vi "Schema Update.vi"(8 "error in (no error)":errorcluster, 10 "Schema":string, 11 "Signal Analysis in":refnum<class "Signal Analysis.lvclass">) -> (0 "error out":errorcluster, 3 "Signal Analysis out":refnum<class "Signal Analysis.lvclass">)   [LabVIEW 2023, in "Data Analysis.lvlib" / "Signal Analysis.lvlib" / "Signal Analysis.lvclass"]
uses:
  Signal Analysis.lvclass
  Signal Analysis.lvclass/Signal Analysis.ctl
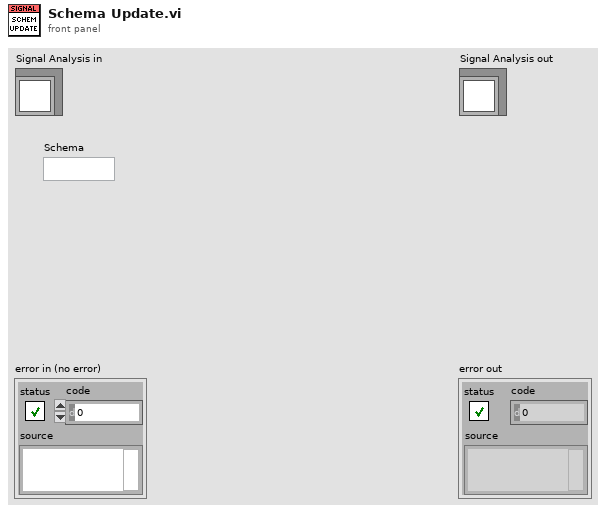
[diagram p1: front panel]
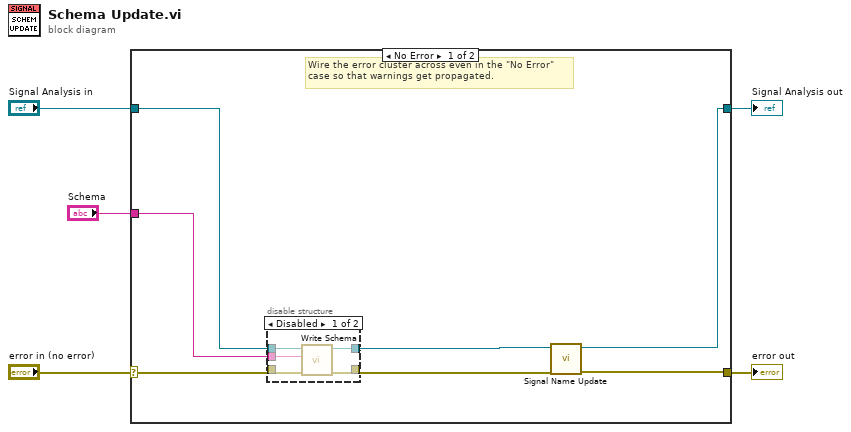
[diagram p0: block diagram]
diagram:
  n1 = case shown="No Error" "error in (no error)" {
    selector: "error in (no error)" -> [w11 w21]
    tunnel: [w6 w21] -> w4
    tunnel: [w8 w20] -> w2
    tunnel: "Signal Analysis in" -> [w12 w20]
    tunnel: "Schema" -> [w10 _]
    frame No Error {
      # "Wire the error cluster across even in the \"No Error\"\ncase so that warnings get propagated."
      n2 = disable-structure shown="Disabled" {
        disable-tunnel: w12 -> [w17 w19]
        disable-tunnel: w11 -> [w16 w18]
        disable-tunnel: w10 -> [w15 _]
        disable-tunnel: [w14 w19] -> w9
        disable-tunnel: [w13 w18] -> w7
        frame Disabled {
          n3 = call "Write Schema.vi"("error in (no error)"=w16, "Schema"=w15, "Signal Analysis in"=w17) -> ("error out"=w13:errorcluster, "Signal Analysis out"=w14:refnum<class "Signal Analysis.lvclass">)  [unwired: 7 in]
        }
        frame Enabled {
        }
      }
      n4 = call "Signal Name Update.vi"("error in (no error)"=w7, "Signal Analysis in"=w9) -> ("error out"=w6:errorcluster, "Signal Analysis out"=w8:refnum<class "Signal Analysis.lvclass">)  [unwired: 8 in]
    }
    frame Error {
    }
  }
  "error out" <- w4
  "Signal Analysis out" <- w2
